vi "Encode String.vi"(10 "String":string, 11 "URI-Component.Query":refnum<class "URI-Component.Query.lvclass">) -> (2 "Encoded String":string)   [LabVIEW 2013, in "openURI.lvlib" / "URI-Component.Query.lvclass"]
uses:
  URI-Component.Query.lvclass
  utilities/isHEXDigit.vi
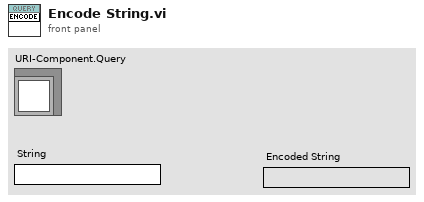
[diagram p1: front panel]
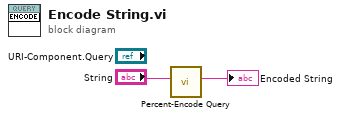
[diagram p0: block diagram]
diagram:
  n1 = call "Percent-Encode Query.vi"("Query"="String") -> ("Pct-Encoded Query"=→"Encoded String":string)  [unwired: 10 in]
